vi "integracao_1.01.vi"() -> ()   [LabVIEW 2011]
panel:
  in  "Numeric":dbl
  out "Boolean 4":bool
  out "appended path":path
  out "String":string
  in  "Arquivo de entrada 2":path=path "\\\\Lidar-database\\LIDAR/data/2005/Ago05/0508"
  out "Array":string[](array[string])
  out "Integral":dbl
  out "pico real":bool
  out "slope negativo":bool
  out "slope positivo":bool
  out "delta tempo menor 0,025":bool
  out "sinal menor que 1":bool
  out "signal 2":dbl
  out "Boolean 3":bool
  out "tempo":dbl
  out "Boolean 2":bool
  out "Waveform Chart 2":dynamicdata(graph)
  out "Boolean":bool
  out "slop curve":dbl
  out "Result":dbl
  out "Waveform Chart":dynamicdata(graph)
  out "signal":dbl
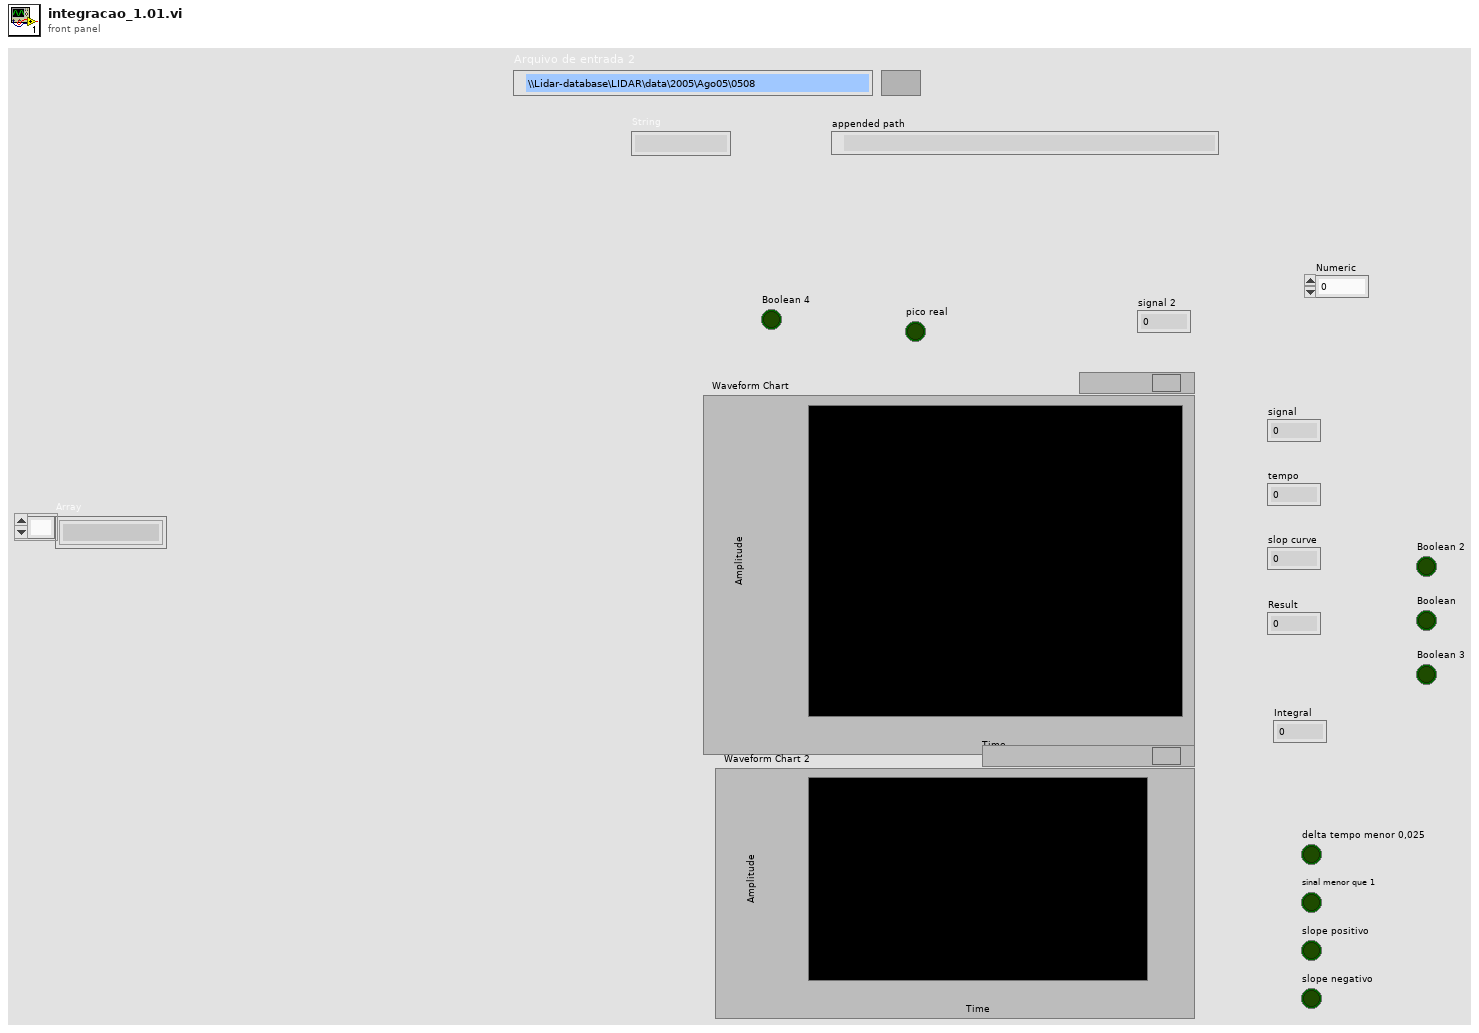
[diagram p1: front panel]
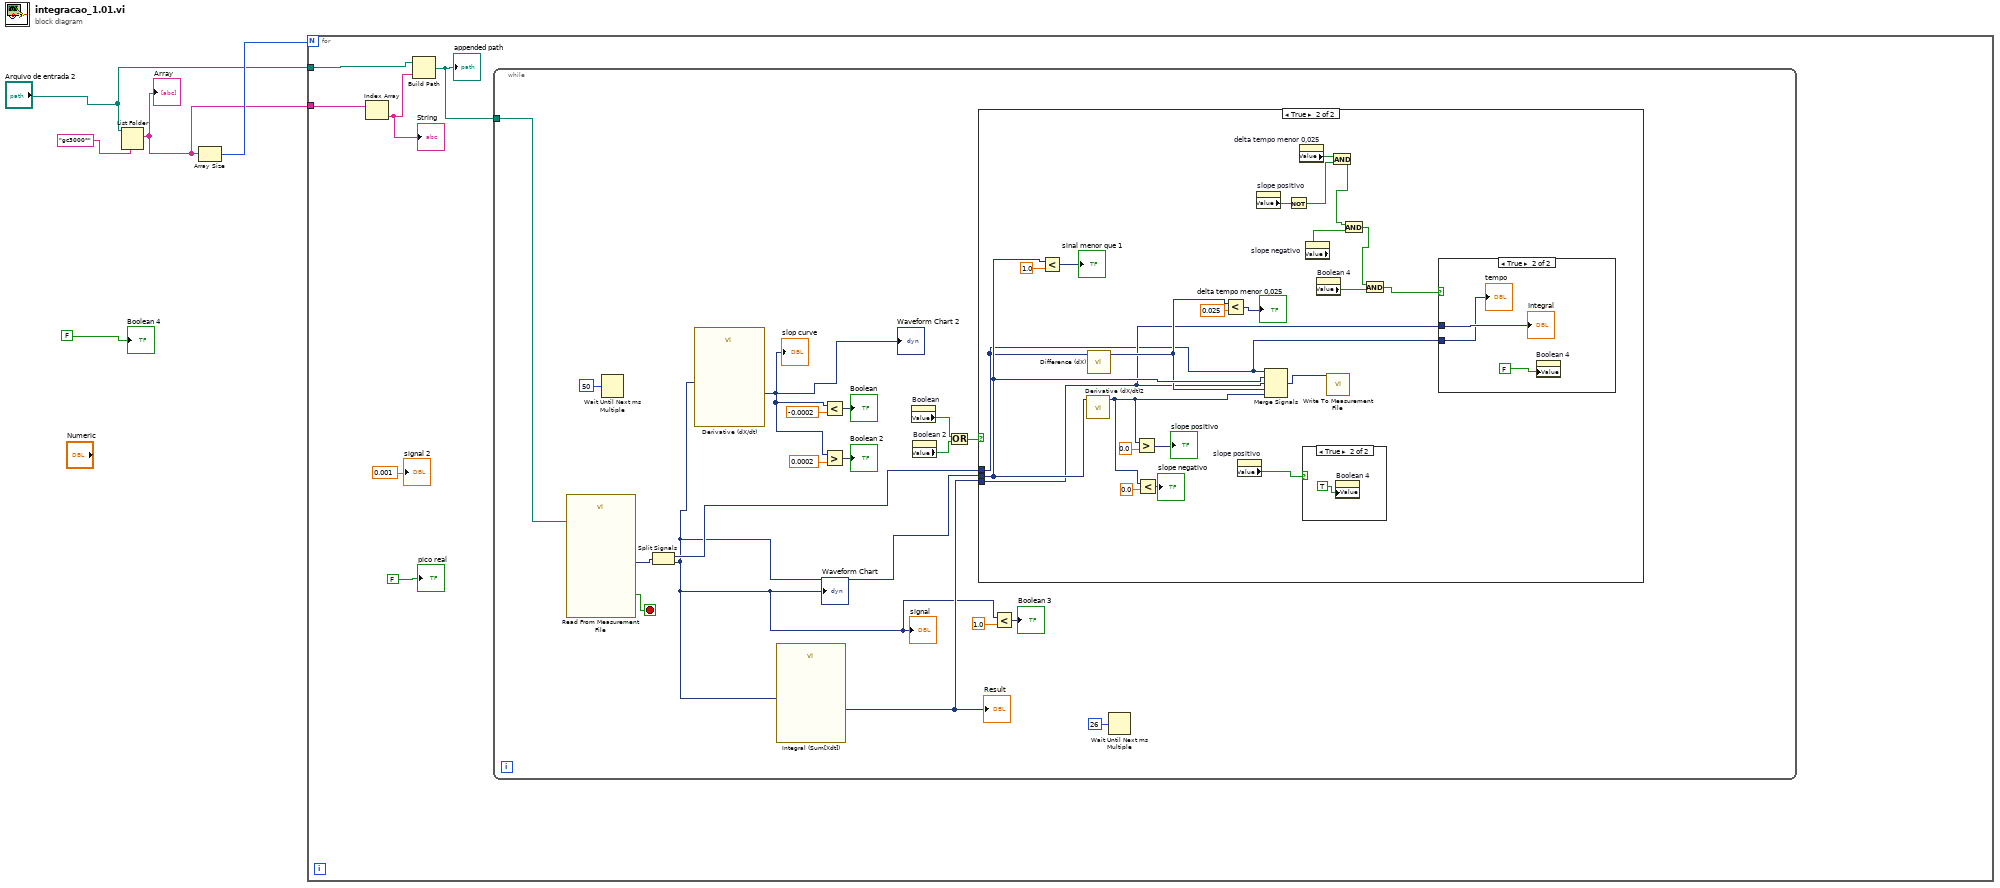
[diagram p0: block diagram]
diagram:
  n1 = List Folder(path="Arquivo de entrada 2", pattern="gc3000*") -> (filenames=w2:string[])  [unwired: 1 in, 4 out]
  "Array" <- w2
  n2 = Array Size(array=w2) -> (size(s)=w4:i32)
  n3 = for {
    N: w4 -> [_]
    tunnel: "Arquivo de entrada 2" -> [w6]
    tunnel: w2 -> [w8]
    n4 = Index Array(array=w8) -> (element=w9:string)  [unwired: 1 in]
    "String" <- w9
    n5 = Build Path(base path=w6, name or relative path=w9) -> (appended path=w7:path)
    "appended path" <- w7
    n6 = while {
      tunnel: w7 -> [w12]
      stop <- w29 stop-if-true
      n7 = call "Read From Measurement File"("Filename"=w12) -> ("Signals"=w23:dynamicdata, "EOF?"=w29:bool)  [unwired: 5 in, 4 out]
      n8 = Wait Until Next ms Multiple(millisecond multiple=u32 50) -> ()  [unwired: 1 out]
      n9 = Split Signals(w23) -> (w22:dynamicdata, w15:dynamicdata)  [unwired: 2 in]
      "signal" <- w15
      "Waveform Chart" <- w15
      n10 = call "Derivative (dX/dt)"("Signals"=w15) -> ("Result"=w13:dynamicdata)  [unwired: 5 in, 1 out]
      "slop curve" <- w13
      "Waveform Chart 2" <- w13
      n11 = call "Integral (Sum[Xdt])"("Signals"=w15) -> ("Result"=w17:dynamicdata)  [unwired: 5 in, 1 out]
      "Result" <- w17
      n12 = Less?(x=w13, y=-0.0002) -> (x < y?=→"Boolean":dynamicdata)
      n13 = Greater?(x=w13, y=0.0002) -> (0:→"Boolean 2":dynamicdata)
      n14 = property on="Boolean" class="Bool (strict)"() -> ("Value"=w20:bool)  [unwired: 2 in, 2 out]
      n15 = property on="Boolean 2" class="Bool (strict)"() -> ("Value"=w19:bool)  [unwired: 2 in, 2 out]
      n16 = Or(x=w20, y=w19) -> (x .or. y?=w18:bool)
      n17 = case shown="True" w18 {
        tunnel: w22 -> [_ w30]
        tunnel: w15 -> [_ w51]
        tunnel: w17 -> [_ w42]
        frame False {
        }
        frame True {
          n18 = Less?(x=w51, y=1.0) -> (x < y?=→"sinal menor que 1":dynamicdata)
          n19 = call "Derivative (dX/dt)2"("Signals"=w51) -> ("Result"=w43:dynamicdata)  [unwired: 5 in, 1 out]
          n20 = call "Difference (dX)"("Signals"=w30) -> ("Result"=w48:dynamicdata)  [unwired: 5 in, 1 out]
          n21 = Greater?(x=w43, y=0.0) -> (0:→"slope positivo":dynamicdata)
          n22 = Less?(x=w43, y=0.0) -> (x < y?=→"slope negativo":dynamicdata)
          n23 = Less?(x=w48, y=0.025) -> (x < y?=→"delta tempo menor 0,025":dynamicdata)
          n24 = property on="slope positivo" class="Bool (strict)"() -> ("Value"=w38:bool)  [unwired: 2 in, 2 out]
          n25 = property on="slope positivo" class="Bool (strict)"() -> ("Value"=w37:bool)  [unwired: 2 in, 2 out]
          n26 = Merge Signals(w30, w51, w42, w48, w43) -> (w52:dynamicdata)
          n27 = Not(x=w37) -> (.not. x?=w36:bool)
          n28 = property on="delta tempo menor 0,025" class="Bool (strict)"() -> ("Value"=w40:bool)  [unwired: 2 in, 2 out]
          n29 = case shown="True" w38 {
            frame False {
            }
            frame True {
              n30 = property on="Boolean 4" class="Bool (strict)"("Value"=TRUE) -> ()  [unwired: 2 in, 2 out]
            }
          }
          n31 = property on="slope negativo" class="Bool (strict)"() -> ("Value"=w35:bool)  [unwired: 2 in, 2 out]
          n32 = property on="Boolean 4" class="Bool (strict)"() -> ("Value"=w31:bool)  [unwired: 2 in, 2 out]
          n33 = call "Write To Measurement File"("Signals"=w52) -> ()  [unwired: 16 in, 3 out]
          n34 = And(x=w40, y=w36) -> (x .and. y?=w34:bool)
          n35 = And(x=w34, y=w35) -> (x .and. y?=w33:bool)
          n36 = And(x=w33, y=w31) -> (x .and. y?=w32:bool)
          n37 = case shown="True" w32 {
            tunnel: w42 -> [_ w56]
            tunnel: w30 -> [_ w54]
            frame False {
            }
            frame True {
              n38 = property on="Boolean 4" class="Bool (strict)"("Value"=FALSE) -> ()  [unwired: 2 in, 2 out]
              "Integral" <- w56
              "tempo" <- w54
            }
          }
        }
      }
      n39 = Less?(x=w15, y=1.0) -> (x < y?=→"Boolean 3":dynamicdata)
      n40 = Wait Until Next ms Multiple(millisecond multiple=u32 26) -> ()  [unwired: 1 out]
    }
    "signal 2" <- 0.001 ("signal 2")
    "pico real" <- FALSE ("pico real")
  }
  "Boolean 4" <- FALSE
